vi "control_elo.vi"(6 "vbus":dbl, 7 "iteration":i32, 8 "error in (no error)":errorcluster, 9 "current time":dbl, 10 "input array":dbl[](array[numeric]), 11 "VISA Refnum in":refnum<visa-resource-name>) -> (0 "error out":errorcluster, 3 "VISA Refnum out":refnum<visa-resource-name>)   [LabVIEW 2019]
uses:
  <instrlib>/Kikusui PLZ 4W Series/Kikusui PLZ 4W Series.lvlib
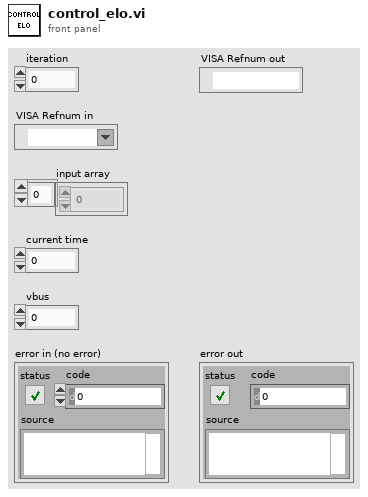
[diagram p1: front panel]
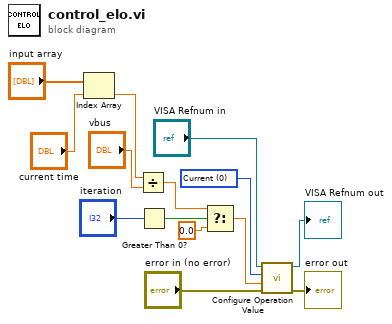
[diagram p0: block diagram]
diagram:
  w1 = u16 0 items=["Current", "Voltage", "Power", "Conductance"] ("Value Type (0:Current)")
  n1 = Index Array(array="input array", index="current time") -> (element=w7:dbl)
  n2 = Divide(x=w7, y="vbus") -> (x/y=w8:dbl)
  n3 = Greater Than 0?(x="iteration") -> (x > 0?=w12:bool)
  n4 = Select(t=w8, s=w12, f=0.0) -> (s? t:f=w9:dbl)
  n5 = call <instrlib>:"Configure Operation Value.vi"("error in (no error)"="error in (no error)", "Values (0)"=w9, "Value Type (0:Current)"=w1, "VISA resource name"="VISA Refnum in") -> ("error out"=→"error out":errorcluster, "VISA resource name out"=→"VISA Refnum out":refnum<visa-resource-name>)  [unwired: 6 in]
